vi "GetExternalInterfaces.vi"(8 "ErrorIn":errorcluster, 11 "ReferenceIn":refnum<class "TraceWindow.lvclass">) -> (0 "ErrorOut":errorcluster, 2 "ExternalInterfaces":T1[](array[typedef]), 3 "ReferenceOut":refnum<class "TraceWindow.lvclass">)   [LabVIEW 2021, in "TraceWindow.lvlib" / "TraceWindow.lvclass"]
uses:
  TraceWindow.lvclass
  Library_TAF_Support/ClusterArrayConversion/BundledArray.ctl
  TraceWindow.lvclass/TraceWindow.ctl
  c918bead-a22c-460a-a6f4-f95520c4e6a6.vi
  Library_TAF_Support/ClusterArrayConversion/ClusterArrayConversion.lvlib
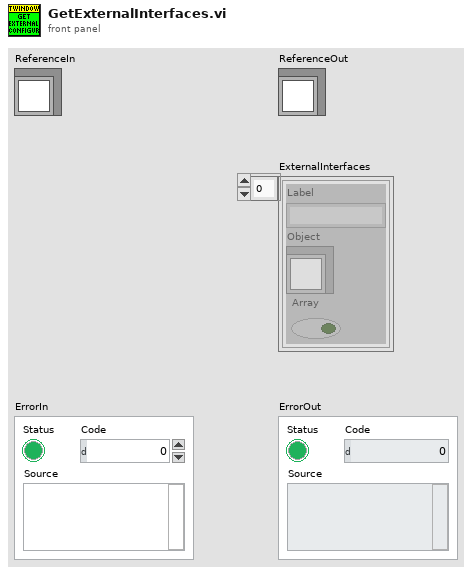
[diagram p1: front panel]
types:
  T1 = typedef "ClusterArrayConversion.lvlib/BundledArray.ctl" = cluster{"Label":string, "Object":refnum<class>, "Array":bool}
  T2 = typedef "TraceWindow.lvlib/TraceWindow.lvclass/ObjectAttributes.ctl" = cluster{"Interfaces":cluster{"Dummys":refnum<class>}, "Locals":cluster{"MainGUIActive":refnum<queue>, "TraceQueue":refnum<queue>}, "Persistent":cluster{"OpenAtClosure":bool, "BufferSize":i32, "Startup":cluster{"OpenAtStartUp":bool, "OpenMinimized":bool}}}
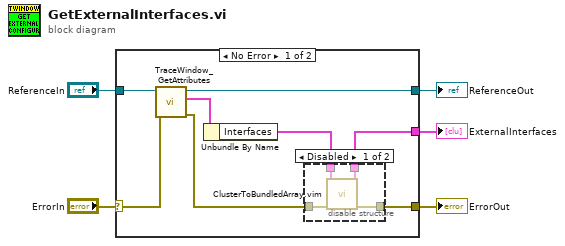
[diagram p0: block diagram]
diagram:
  n1 = case shown="No Error" "ErrorIn" {
    selector: "ErrorIn" -> [w13 w19]
    tunnel: [w11 w19] -> w4
    tunnel: [w8 w18] -> w2
    tunnel: "ReferenceIn" -> [w9 w18]
    tunnel: [w6 _] -> w1
    frame No Error {
      n2 = call "TraceWindow_GetAttributes.vi"("ErrorIn"=w13, "ReferenceIn"=w9) -> ("ErrorOut"=w12:errorcluster, "Data"=w10:T2, "ReferenceOut"=w8:refnum<class "TraceWindow.lvclass">)  [unwired: 6 in, 1 out]
      n3 = Unbundle By Name(w10) -> ("Interfaces"=w7:cluster{"Dummys":refnum<class>})
      n4 = disable-structure shown="Disabled" {
        disable-tunnel: w12 -> [w17 _]
        disable-tunnel: w7 -> [w15 _]
        disable-tunnel: [w14 _] -> w6
        disable-tunnel: [w16 _] -> w11
        frame Disabled {
          n5 = call "ClusterToBundledArray.vim"("ErrorIn"=w17, "Interfaces"=w15) -> ("ErrorOut"=w16:errorcluster, "BundeledLabels"=w14:T1[])  [unwired: 8 in]
        }
        frame Enabled {
        }
      }
    }
    frame Error {
    }
  }
  "ErrorOut" <- w4
  "ReferenceOut" <- w2
  "ExternalInterfaces" <- w1
